vi "Membrane wash timer.vi"(2 "УЗ7":dbl format="%#_13g", 5 "СЧ2":dbl) -> (19 "Status":bool, 20 "Насос 3":bool=TRUE, 21 "КР5":dbl format="%#_13g", 22 "КР6":dbl format="%#_13g", 23 "КР7":dbl format="%#_13g", 24 "КР4":dbl format="%#_13g", 25 "КР8":dbl format="%#_13g", 26 "Насос 8":bool=TRUE, 27 "Error output":bool)   [LabVIEW 2019]
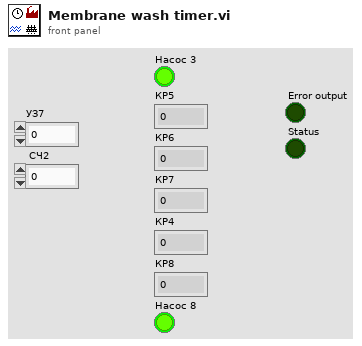
[diagram p1: front panel]
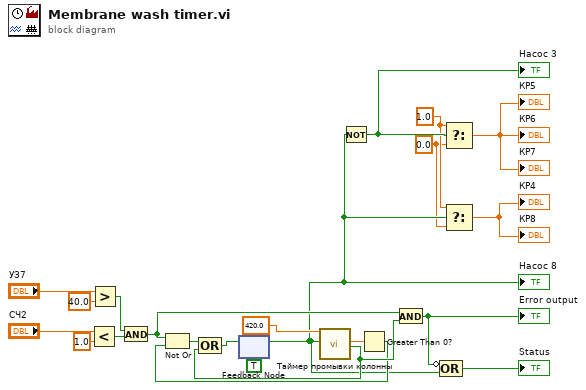
[diagram p0: block diagram]
diagram:
  w3 = 1.0
  w2 = 0.0
  n1 = Less?(x="СЧ2", y=1.0) -> (x < y?=w11:bool)
  n2 = Greater?(x="УЗ7", y=40.0) -> (0:w9:bool)
  n3 = And(x=w9, y=w11) -> (x .and. y?=w10:bool)
  n4 = feedback #1(TRUE) -> (w4:bool)
  "Насос 8" <- w4
  n5 = call "Таймер промывки колонны"("Time Target (s)"=420.0, "Reset"=w4) -> ("Elapsed Time (s)"=w17:dbl, "Time has Elapsed"=w21:bool)  [unwired: 10 in, 6 out]
  n6 = Not(x=w4) -> (.not. x?=w6:bool)
  "Насос 3" <- w6
  n7 = Greater Than 0?(x=w17) -> (x > 0?=w19:bool)
  n8 = Not Or(1:w19, 2:w10) -> (0:w20:bool)
  n9 = Compound Arithmetic op=OR(w20, w21) -> (w22:bool)
  n10 = feedback-in #1(w22) -> ()
  n11 = And(x=w10, y=w21) -> (x .and. y?=w8:bool)
  "Error output" <- w8
  n12 = Compound Arithmetic op=OR(invert w8, w4) -> (→"Status":bool)
  n13 = Select(t=w3, s=w6, f=w2) -> (s? t:f=→"КР5" →"КР6" →"КР7":dbl)
  n14 = Select(t=w3, s=w4, f=w2) -> (s? t:f=→"КР4" →"КР8":dbl)
